vi "Convert Diagnostic ERD for Display.vi"(8 "Error In":errorcluster, 11 "Heater Diag.":u32) -> (0 "Error Out":errorcluster, 3 "String":string)   [LabVIEW 2016]
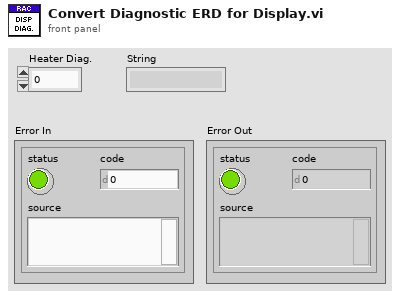
[diagram p1: front panel]
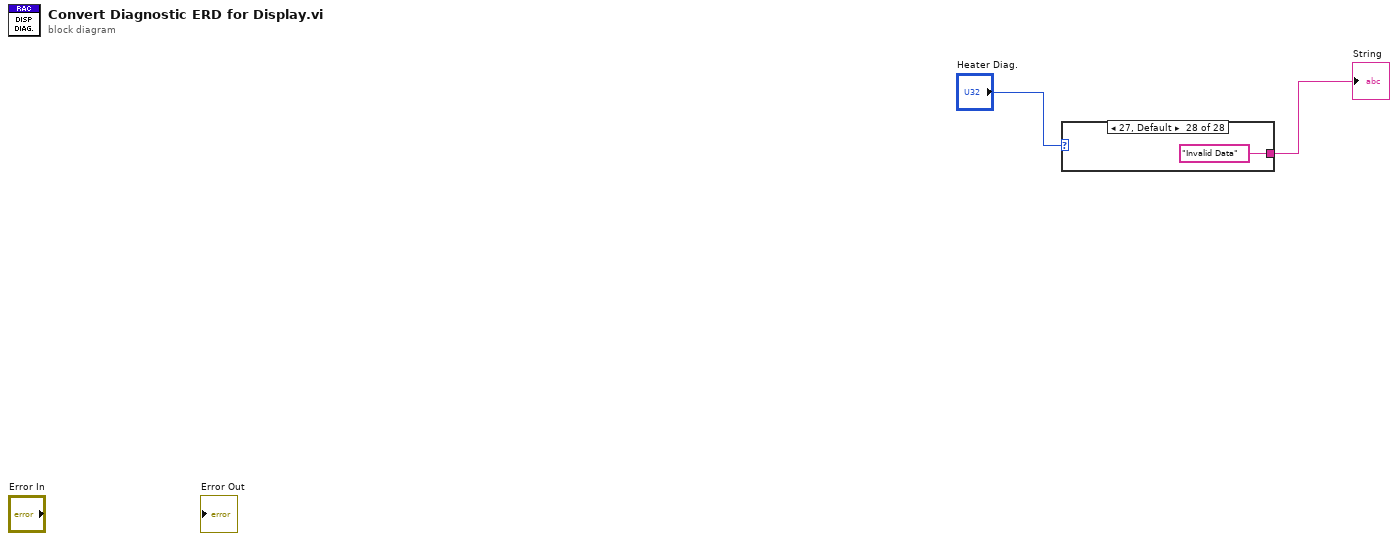
[diagram p0: block diagram]
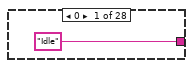
[diagram p2: hidden frame]
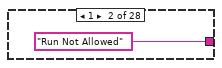
[diagram p3: hidden frame]
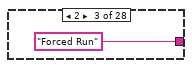
[diagram p4: hidden frame]
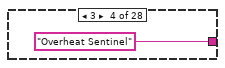
[diagram p5: hidden frame]
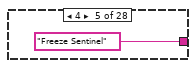
[diagram p6: hidden frame]
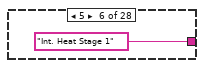
[diagram p7: hidden frame]
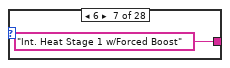
[diagram p8: hidden frame]
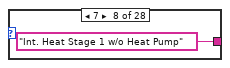
[diagram p9: hidden frame]
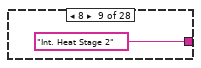
[diagram p10: hidden frame]
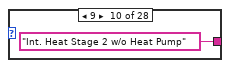
[diagram p11: hidden frame]
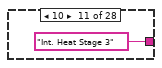
[diagram p12: hidden frame]
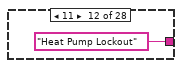
[diagram p13: hidden frame]
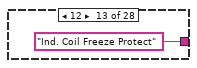
[diagram p14: hidden frame]
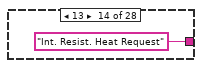
[diagram p15: hidden frame]
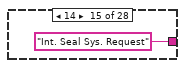
[diagram p16: hidden frame]
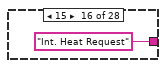
[diagram p17: hidden frame]
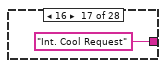
[diagram p18: hidden frame]
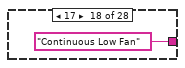
[diagram p19: hidden frame]
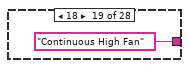
[diagram p20: hidden frame]
diagram:
  n1 = case shown="27, Default" "Heater Diag." {
    tunnel: ["Idle" "Run Not Allowed" "Forced Run" "Overheat Sentinel" "Freeze Sentinel" "Int. Heat Stage 1" "Int. Heat Stage 1 w/Forced Boost" "Int. Heat Stage 1 w/o Heat Pump" "Int. Heat Stage 2" "Int. Heat Stage 2 w/o Heat Pump" "Int. Heat Stage 3" "Heat Pump Lockout" "Ind. Coil Freeze Protect" "Int. Resist. Heat Request" "Int. Seal Sys. Request" "Int. Heat Request" "Int. Cool Request" "Continuous Low Fan" "Continuous High Fan" "Fan Pulsing" "Fan Only User Mode Setting" "Ext. Thermostat" "Remote Control" "Defrost" "Central Desk Lockout" "Fault" "QuickHeatRecovery" "Invalid Data"] -> w2
    frame 0 {
    }
    frame 1 {
    }
    frame 2 {
    }
    frame 3 {
    }
    frame 4 {
    }
    frame 5 {
    }
    frame 6 {
    }
    frame 7 {
    }
    frame 8 {
    }
    frame 9 {
    }
    frame 10 {
    }
    frame 11 {
    }
    frame 12 {
    }
    frame 13 {
    }
    frame 14 {
    }
    frame 15 {
    }
    frame 16 {
    }
    frame 17 {
    }
    frame 18 {
    }
    frame 19 {
    }
    frame 20 {
    }
    frame 21 {
    }
    frame 22 {
    }
    frame 23 {
    }
    frame 24 {
    }
    frame 25 {
    }
    frame 26 {
    }
    frame 27, Default {
    }
  }
  "String" <- w2
